vi "Import_xy-wiArray.vi"(5 "InputArray":dbl[][](array[numeric]) format="%0.3f", 7 "Uniform":bool) -> (0 "XY Full":cluster{dbl, dbl}[](array[cluster]), 1 "XY Unique":cluster{"X Unique":dbl[], "Y Unique":dbl[]}, 2 "Wavelength":dbl[](array[numeric]), 3 "Intensity":dbl[][](array[numeric]), 4 "XY Full Interpol.":cluster{dbl, dbl}[](array[cluster]), 6 "Axes":T1)   [LabVIEW 2010]
uses:
  <vilib>/Analysis/polynomials.llb/Unique Numbers and Multiplicity (DBL).vi
  <vilib>/Analysis/NI_AALPro.lvlib
  <vilib>/Analysis/NI_AALBase.lvlib
panel:
  # "Imports a 2D-array containing XY-WI data. XY varies over columns, XY-data are stored in the first two rows, respctively.\nW (wavelength/Raman shift) varies over rows."
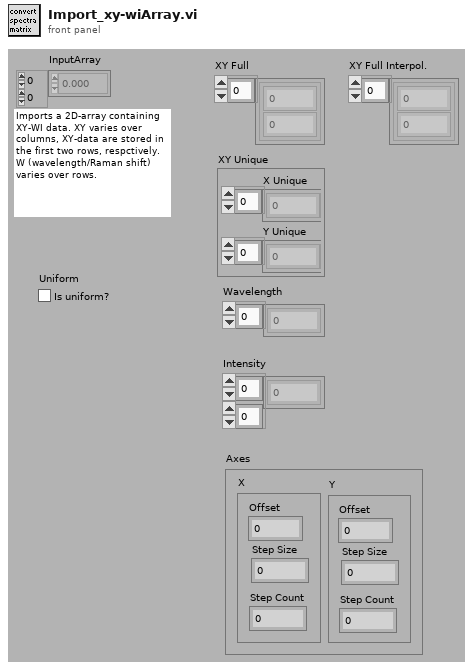
[diagram p1: front panel]
types:
  T1 = cluster{"X":cluster{"Offset":dbl, "Step Size":dbl, "Step Count":i32}, "Y":cluster{"Offset":dbl, "Step Size":dbl, "Step Count":i32}}
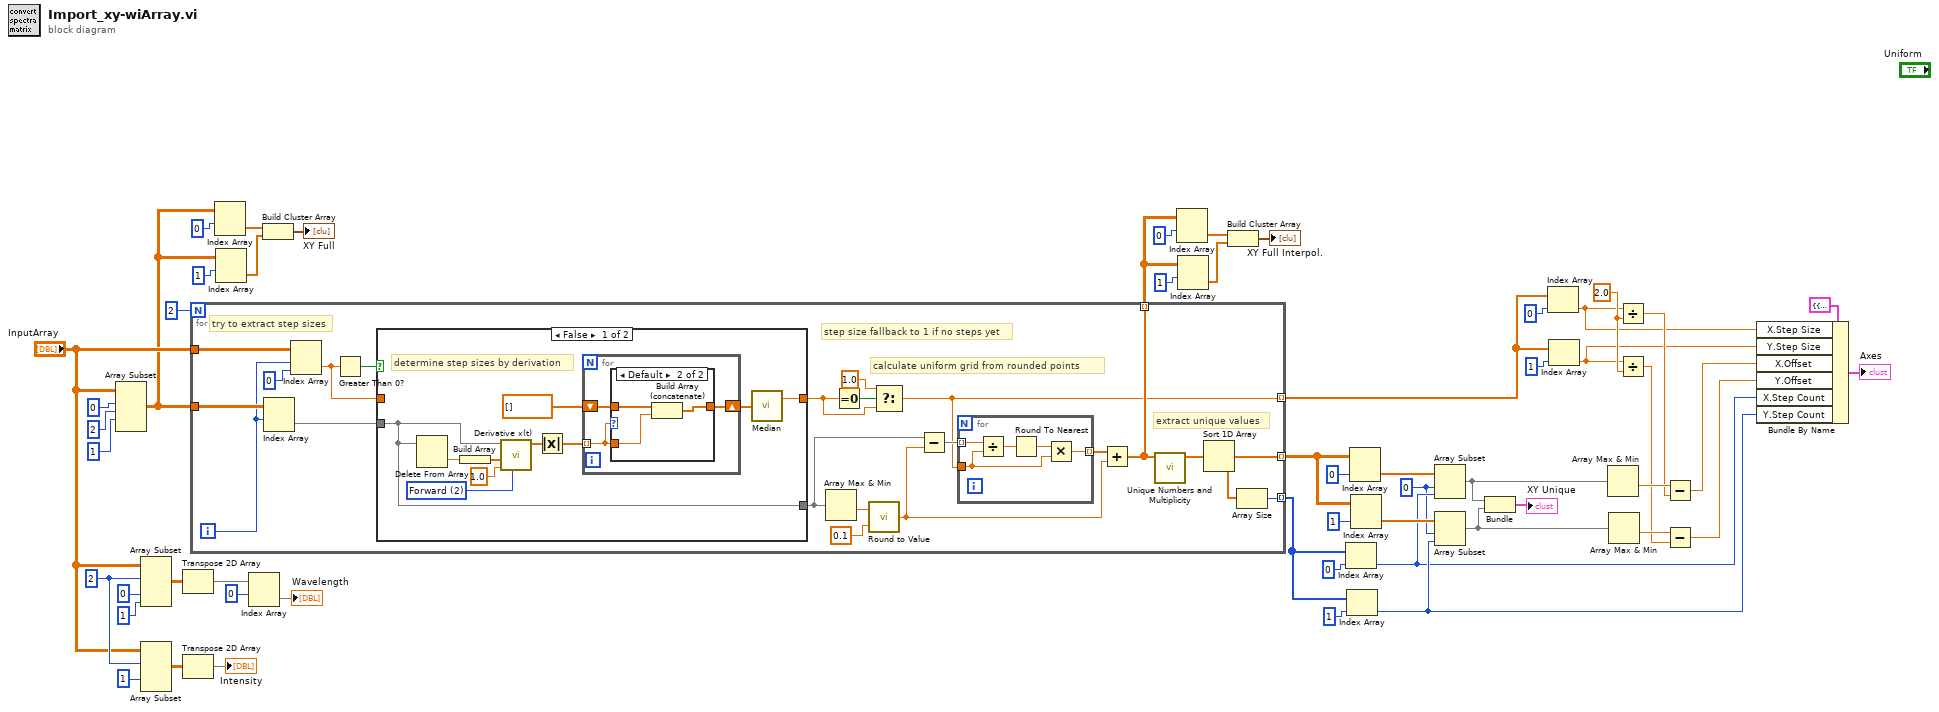
[diagram p0: block diagram]
diagram:
  w2 = 0 ("index (row)")
  w21 = 2.0 ("y")
  w51 = 2 ("Index")
  n1 = Array Subset(array="InputArray", index (row)=0 ("Index"), length (row)=2 ("Länge"), index (col)=1 ("Index")) -> (w33:dbl[][])  [unwired: 1 in]
  n2 = Array Subset(array="InputArray", index (row)=w51, index (col)=0 ("Index"), length (col)=1 ("Länge")) -> (w48:dbl[][])  [unwired: 1 in]
  n3 = Array Subset(array="InputArray", index (row)=w51, index (col)=1 ("Index")) -> (w46:dbl[][])  [unwired: 2 in]
  n4 = Transpose 2D Array(2D array=w48) -> (transposed array=w47:dbl[][])
  n5 = Transpose 2D Array(2D array=w46) -> (transposed array=→"Intensity":dbl[][])
  n6 = for {
    N: 2 -> [_]
    tunnel: "InputArray" -> [w75]
    tunnel: w33 -> [w73]
    tunnel: [w67] -> w28 mode=indexing
    tunnel: [w60] -> w7 mode=indexing
    tunnel: [w62] -> w23 mode=indexing
    tunnel: [w59] -> w12 mode=indexing
    i -> [w65]
    # "step size fallback to 1 if no steps yet"
    # "extract unique values"
    # "calculate uniform grid from rounded points"
    # "try to extract step sizes"
    n7 = Index Array(array=w73, index (row)=w65) -> (element=w72:dbl[])  [unwired: 1 in]
    n8 = Index Array(array=w75, index (row)=w65, index (col)=0 ("disabled index (col)")) -> (element=w71:dbl)
    n9 = Greater Than 0?(x=w71) -> (x > 0?=w74:bool)
    n10 = case shown="False" w74 {
      tunnel: w72 -> [w82 w100]
      tunnel: [w83 w99] -> w63
      tunnel: [w82 w100] -> w69
      tunnel: w71 -> [_ w99]
      frame False {
        w89 = u16 2 items=["2nd Order Central", "4th Order Central", "Forward", "Backward"] ("method")
        # "determine step sizes by derivation"
        n11 = Delete From Array(array=w82) -> (deleted portion=w90:dbl)  [unwired: 2 in, 1 out]
        n12 = Build Array(w90) -> (w91:dbl[])
        n13 = call <vilib>:"Derivative x(t).vi"("method"=w89, "dt"=1.0, "Final Condition"=w91, "X"=w82) -> ("dX/dt"=w86:dbl[])  [unwired: 6 in, 1 out]
        n14 = Absolute Value(x=w86) -> (abs(x)=w85:dbl[])
        n15 = for {
          shift-right: [w93] -> w84
          shift-left: dbl[] [] ("abs(x)") -> [w94]
          tunnel: w85 -> [w92] mode=indexing
          n16 = case shown="Default" w92 {
            tunnel: w94 -> [w95 w98]
            tunnel: [w95 w97] -> w93
            tunnel: w92 -> [_ w96]
            frame 0 {
            }
            frame Default {
              n17 = Build Array (concatenate)(w98, w96) -> (w97:dbl[])
            }
          }
        }
        n18 = call <vilib>:"Median.vi"("X"=w84) -> ("median"=w83:dbl)  [unwired: 1 out]
      }
      frame True {
        # "step sizes were already determines"
      }
    }
    n19 = Array Max & Min(array=w69) -> (min value=w56:dbl)  [unwired: 3 out]
    n20 = Equal To 0?(x=w63) -> (x = 0?=w64:bool)
    n21 = call "Round to Value.vi"("Precision"=0.1, "Value In"=w56) -> ("Rounded"=w58:dbl)
    n22 = Select(t=1.0, s=w64, f=w63) -> (s? t:f=w62:dbl)
    n23 = Subtract(x=w69, y=w58) -> (x-y=w70:dbl[])
    n24 = for {
      tunnel: w70 -> [w80] mode=indexing
      tunnel: w62 -> [w78]
      tunnel: [w77] -> w68 mode=indexing
      n25 = Divide(x=w80, y=w78) -> (x/y=w81:dbl)
      n26 = Round To Nearest(number=w81) -> (nearest integer value=w79:dbl)
      n27 = Multiply(x=w79, y=w78) -> (x*y=w77:dbl)
    }
    n28 = Add(x=w68, y=w58) -> (x+y=w67:dbl[])
    n29 = call-poly <vilib>:"Unique Numbers and Multiplicity.vi"("Numbers"=w67) -> ("Unique Numbers"=w66:dbl[])  [unwired: 8 in, 2 out]
    n30 = Sort 1D Array(array=w66) -> (sorted array=w60:dbl[])
    n31 = Array Size(array=w60) -> (size(s)=w59:i32)
  }
  n32 = Index Array(array=w33, index (row)=0) -> (element=w32:dbl[])  [unwired: 1 in]
  n33 = Index Array(array=w33, index (row)=1) -> (element=w31:dbl[])  [unwired: 1 in]
  n34 = Index Array(array=w47, index (row)=0 ("Index")) -> (element=→"Wavelength":dbl[])  [unwired: 1 in]
  n35 = Build Cluster Array(w32, w31) -> (→"XY Full":cluster{dbl, dbl}[])
  n36 = Index Array(array=w28, index (row)=0) -> (element=w26:dbl[])  [unwired: 1 in]
  n37 = Index Array(array=w28, index (row)=1) -> (element=w27:dbl[])  [unwired: 1 in]
  n38 = Build Cluster Array(w26, w27) -> (→"XY Full Interpol.":cluster{dbl, dbl}[])
  n39 = Index Array(array=w12, index=0 ("index (row)")) -> (element=w3:i32)
  n40 = Index Array(array=w12, index=1 ("index (row)")) -> (element=w4:i32)
  n41 = Index Array(array=w7, index (row)=0) -> (element=w6:dbl[])  [unwired: 1 in]
  n42 = Index Array(array=w7, index (row)=1) -> (element=w5:dbl[])  [unwired: 1 in]
  n43 = Array Subset(array=w6, index=w2, length=w3) -> (w11:dbl[])
  n44 = Array Subset(array=w5, index=w2, length=w4) -> (w10:dbl[])
  n45 = Bundle(w11, w10) -> (→"XY Unique":cluster{dbl[], dbl[]})  [unwired: 1 in]
  n46 = Index Array(array=w23, index=0 ("index (row)")) -> (element=w20:dbl)
  n47 = Index Array(array=w23, index=1 ("index (row)")) -> (element=w19:dbl)
  n48 = Array Max & Min(array=w11) -> (min value=w38:dbl)  [unwired: 3 out]
  n49 = Array Max & Min(array=w10) -> (min value=w17:dbl)  [unwired: 3 out]
  n50 = Divide(x=w20, y=w21) -> (x/y=w22:dbl)
  n51 = Divide(x=w19, y=w21) -> (x/y=w16:dbl)
  n52 = Subtract(x=w38, y=w22) -> (x-y=w18:dbl)
  n53 = Subtract(x=w17, y=w16) -> (x-y=w15:dbl)
  n54 = Bundle By Name(cluster=T1 {"X"={"Offset"=0.0, "Step Size"=0.0, "Step Count"=0}, "Y"={"Offset"=0.0, "Step Size"=0.0, "Step Count"=0}} ("Axes"), "X.Step Size"=w20, "Y.Step Size"=w19, "X.Offset"=w18, "Y.Offset"=w15, "X.Step Count"=w3, "Y.Step Count"=w4) -> (→"Axes":T1)
